vi "Is System Running Check.vi"(3 "error in (no error)":errorcluster, 4 "connect timeout in ms (4s)":u32=4000, 5 "IP Address":string="10.0.42.155") -> (0 "error out":errorcluster, 2 "x = y?":bool)   [LabVIEW 2013]
uses:
  <vilib>/nisyscfg/Initialize (String).vi
  <vilib>/nisyscfg/Close (System).vi
  <vilib>/nisyscfg/nisyscfg.lvlib
  <resource>/objmgr/nisysapi.rc
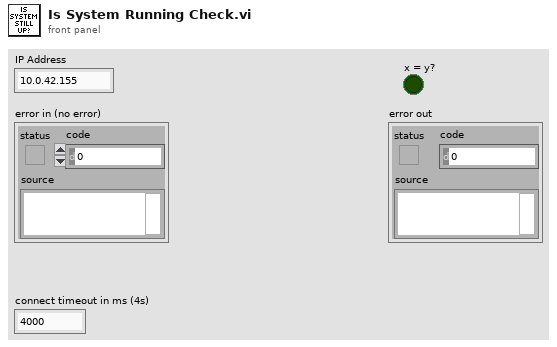
[diagram p1: front panel]
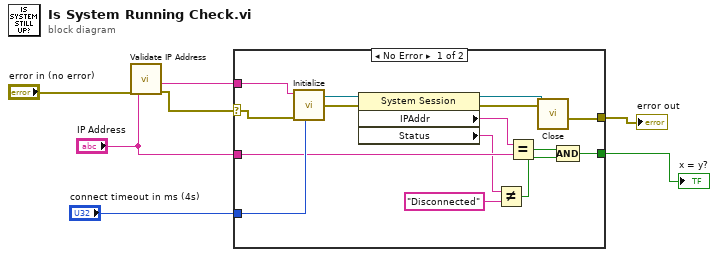
[diagram p0: block diagram]
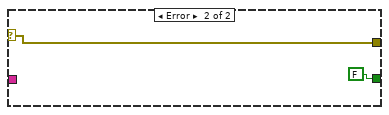
[diagram p2: hidden frame]
diagram:
  n1 = call "Validate IP Address.vi"("Error In"="error in (no error)", "IP Address"="IP Address") -> ("Error Out"=w6:errorcluster, "IP Address Out"=w5:string)  [unwired: 4 in]
  n2 = case shown="No Error" w6 {
    selector: w6 -> [w20 w24]
    tunnel: w5 -> [w19 _]
    tunnel: [w16 w24] -> w4
    tunnel: "connect timeout in ms (4s)" -> [w18 _]
    tunnel: "IP Address" -> [w13 _]
    tunnel: [w8 FALSE] -> w1
    frame No Error {
      n3 = call-poly <vilib>:"Initialize.vi"("connect timeout in ms (4s)"=w18, "error in (no error)"=w20, "target (localhost)"=w19) -> ("error out"=w21:errorcluster, "session out"=w22:refnum<k21>)  [unwired: 6 in, 1 out]
      n4 = property class="System Session"(reference=w22, error in=w21) -> (reference out=w15:refnum<k21>, error out=w17:errorcluster, "IPAddr"=w14:string, "Status"=w11:string)
      n5 = Not Equal?(x=w11, y="Disconnected") -> (x != y?=w9:bool)
      n6 = Equal?(x=w14, y=w13) -> (x = y?=w10:bool)
      n7 = call-poly <vilib>:"Close.vi"("error in (no error)"=w17, "session in"=w15) -> ("error out"=w16:errorcluster)  [unwired: 9 in]
      n8 = Compound Arithmetic op=AND(w10, w9) -> (w8:bool)
    }
    frame Error {
    }
  }
  "error out" <- w4
  "x = y?" <- w1
